vi "Test Write Strings.vi"(11 "TwinCAT ADS in":refnum<class "TwinCAT ADS.lvclass">) -> (3 "TwinCAT ADS out":refnum<class "TwinCAT ADS.lvclass">)   [LabVIEW 2018]
uses:
  TwinCAT ADS Class/TwinCAT ADS.lvclass
  f519b359-897f-4db4-aefa-8844a362c035.vi
  6c1bdafb-d09a-46e8-b3f2-64a16ab2d4cb.vi
  40482fa9-f387-4bff-83e3-c0961ce42c5b.vi
  3bee3f50-b92d-484c-8fb5-3521a61bfde1.vi
  67abcce4-d906-4956-a77e-4a47c9dde040.vi
  c0c5b84e-43cd-4ba1-b01f-cca28dc7bea8.vi
  903064a7-6281-4536-8159-57f8726da337.vi
  a8d287bd-4485-4814-8cd1-9655769c98e5.vi
  TwinCAT ADS Class/VIs/Data/Read.vi
  <vilib>/addons/_JKI Toolkits/Caraya/classes/Assert/Assert Equal Value and Type_Variant.vi
  <vilib>/addons/_JKI Toolkits/Caraya/classes/Test/Test.lvclass
  <vilib>/addons/_JKI Toolkits/Caraya/classes/Assert/Assert.lvclass
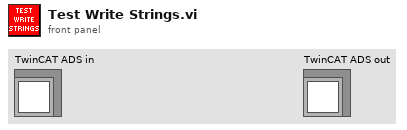
[diagram p1: front panel]
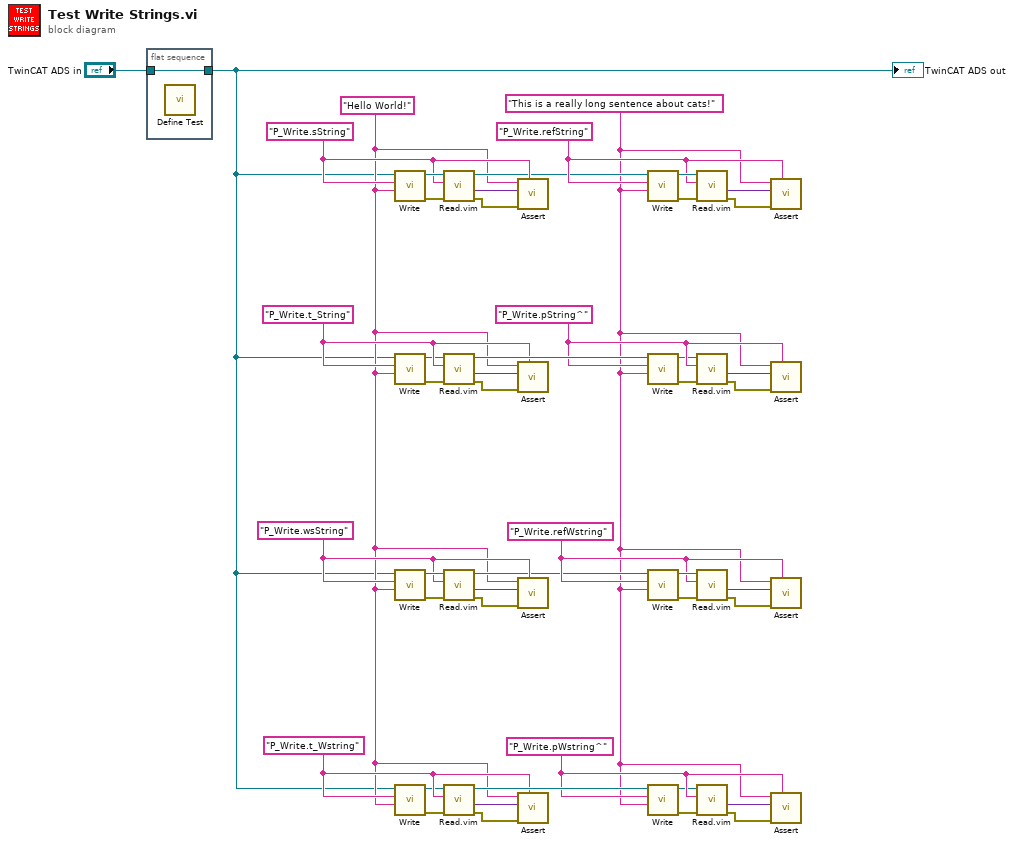
[diagram p0: block diagram]
diagram:
  w13 = "P_Write.pWstring^" ("Symbol Name")
  w8 = "P_Write.t_Wstring" ("Symbol Name")
  w16 = "P_Write.refWstring" ("Symbol Name")
  w21 = "P_Write.wsString" ("Symbol Name")
  w35 = "P_Write.pString^" ("Symbol Name")
  w30 = "P_Write.t_String" ("Symbol Name")
  w3 = "This is a really long sentence about cats!" ("Symbol Name")
  w2 = "Hello World!" ("Symbol Name")
  w38 = "P_Write.refString" ("Symbol Name")
  w43 = "P_Write.sString" ("Symbol Name")
  n1 = flat-sequence {
    tunnel: "TwinCAT ADS in" -> [w49]
    tunnel: [w49] -> w1
    frame #0 {
      n2 = call <vilib>:"Define Test.vi"() -> ()  [unwired: 10 in, 2 out]
    }
  }
  n3 = call "Write.vi"("Value"=w2, "Symbol Name"=w43, "TwinCAT ADS in"=w1) -> ("error out"=w46:errorcluster, "TwinCAT ADS out"=w47:refnum<class "TwinCAT ADS.lvclass">)  [unwired: 7 in]
  n4 = call "Write.vi"("Value"=w2, "Symbol Name"=w30, "TwinCAT ADS in"=w1) -> ("error out"=w27:errorcluster, "TwinCAT ADS out"=w26:refnum<class "TwinCAT ADS.lvclass">)  [unwired: 7 in]
  n5 = call "Write.vi"("Value"=w2, "Symbol Name"=w21, "TwinCAT ADS in"=w1) -> ("error out"=w24:errorcluster, "TwinCAT ADS out"=w25:refnum<class "TwinCAT ADS.lvclass">)  [unwired: 7 in]
  n6 = call "Write.vi"("Value"=w2, "Symbol Name"=w8, "TwinCAT ADS in"=w1) -> ("error out"=w5:errorcluster, "TwinCAT ADS out"=w4:refnum<class "TwinCAT ADS.lvclass">)  [unwired: 7 in]
  n7 = call "Read.vim"("error in (no error)"=w46, "Symbol Name"=w43, "TwinCAT ADS in"=w47) -> ("error out"=w45:errorcluster, "Value"=w44:variant, "TwinCAT ADS out"=w37:refnum<class "TwinCAT ADS.lvclass">)  [unwired: 6 in]
  n8 = call "Read.vim"("error in (no error)"=w27, "Symbol Name"=w30, "TwinCAT ADS in"=w26) -> ("error out"=w28:errorcluster, "Value"=w29:variant, "TwinCAT ADS out"=w36:refnum<class "TwinCAT ADS.lvclass">)  [unwired: 6 in]
  n9 = call "Read.vim"("error in (no error)"=w24, "Symbol Name"=w21, "TwinCAT ADS in"=w25) -> ("error out"=w23:errorcluster, "Value"=w22:variant, "TwinCAT ADS out"=w15:refnum<class "TwinCAT ADS.lvclass">)  [unwired: 6 in]
  n10 = call "Read.vim"("error in (no error)"=w5, "Symbol Name"=w8, "TwinCAT ADS in"=w4) -> ("error out"=w6:errorcluster, "Value"=w7:variant, "TwinCAT ADS out"=w14:refnum<class "TwinCAT ADS.lvclass">)  [unwired: 6 in]
  n11 = call-poly <vilib>:"Assert.vi"("Label"=w43, "error in (no error)"=w45, "Y"=w44, "X"=w2) -> ()  [unwired: 6 in, 2 out]
  n12 = call-poly <vilib>:"Assert.vi"("Label"=w30, "error in (no error)"=w28, "Y"=w29, "X"=w2) -> ()  [unwired: 6 in, 2 out]
  n13 = call-poly <vilib>:"Assert.vi"("Label"=w21, "error in (no error)"=w23, "Y"=w22, "X"=w2) -> ()  [unwired: 6 in, 2 out]
  n14 = call-poly <vilib>:"Assert.vi"("Label"=w8, "error in (no error)"=w6, "Y"=w7, "X"=w2) -> ()  [unwired: 6 in, 2 out]
  n15 = call "Write.vi"("Value"=w3, "Symbol Name"=w38, "TwinCAT ADS in"=w37) -> ("error out"=w41:errorcluster, "TwinCAT ADS out"=w42:refnum<class "TwinCAT ADS.lvclass">)  [unwired: 7 in]
  n16 = call "Write.vi"("Value"=w3, "Symbol Name"=w35, "TwinCAT ADS in"=w36) -> ("error out"=w32:errorcluster, "TwinCAT ADS out"=w31:refnum<class "TwinCAT ADS.lvclass">)  [unwired: 7 in]
  n17 = call "Write.vi"("Value"=w3, "Symbol Name"=w16, "TwinCAT ADS in"=w15) -> ("error out"=w19:errorcluster, "TwinCAT ADS out"=w20:refnum<class "TwinCAT ADS.lvclass">)  [unwired: 7 in]
  n18 = call "Write.vi"("Value"=w3, "Symbol Name"=w13, "TwinCAT ADS in"=w14) -> ("error out"=w10:errorcluster, "TwinCAT ADS out"=w9:refnum<class "TwinCAT ADS.lvclass">)  [unwired: 7 in]
  n19 = call "Read.vim"("error in (no error)"=w41, "Symbol Name"=w38, "TwinCAT ADS in"=w42) -> ("error out"=w40:errorcluster, "Value"=w39:variant)  [unwired: 6 in, 1 out]
  n20 = call "Read.vim"("error in (no error)"=w32, "Symbol Name"=w35, "TwinCAT ADS in"=w31) -> ("error out"=w33:errorcluster, "Value"=w34:variant)  [unwired: 6 in, 1 out]
  n21 = call "Read.vim"("error in (no error)"=w19, "Symbol Name"=w16, "TwinCAT ADS in"=w20) -> ("error out"=w18:errorcluster, "Value"=w17:variant)  [unwired: 6 in, 1 out]
  n22 = call "Read.vim"("error in (no error)"=w10, "Symbol Name"=w13, "TwinCAT ADS in"=w9) -> ("error out"=w11:errorcluster, "Value"=w12:variant)  [unwired: 6 in, 1 out]
  n23 = call-poly <vilib>:"Assert.vi"("Label"=w38, "error in (no error)"=w40, "Y"=w39, "X"=w3) -> ()  [unwired: 6 in, 2 out]
  n24 = call-poly <vilib>:"Assert.vi"("Label"=w35, "error in (no error)"=w33, "Y"=w34, "X"=w3) -> ()  [unwired: 6 in, 2 out]
  n25 = call-poly <vilib>:"Assert.vi"("Label"=w16, "error in (no error)"=w18, "Y"=w17, "X"=w3) -> ()  [unwired: 6 in, 2 out]
  n26 = call-poly <vilib>:"Assert.vi"("Label"=w13, "error in (no error)"=w11, "Y"=w12, "X"=w3) -> ()  [unwired: 6 in, 2 out]
  "TwinCAT ADS out" <- w1
